vi "set print interval.vi"(4 "error in (no error)":errorcluster, 5 "auto/manual":bool, 6 "seconds/data point":u16=1 min=1 max=9999 step=1) -> (0 "error out":errorcluster, 2 "seconds/data point":u16=1 min=1 max=9999 step=1)   [LabVIEW 2010]
uses:
  serial commands.ctl
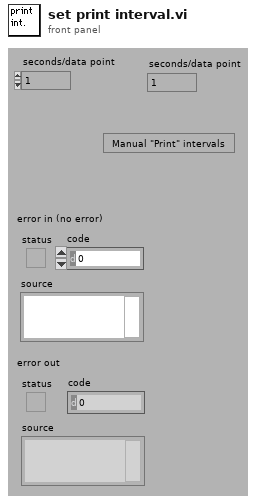
[diagram p1: front panel]
types:
  T1 = typedef "serial commands.ctl" = enum16{"configure", "VISA resource", "write line", "read line", "Clear buffer", "close"}
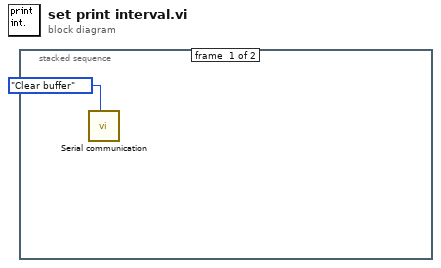
[diagram p0: block diagram]
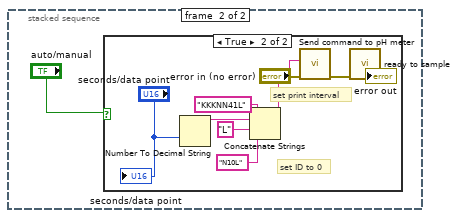
[diagram p2: hidden frame]
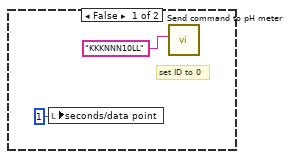
[diagram p3: hidden frame]
diagram:
  n1 = stacked-sequence {
    frame #0 {
      n2 = call <userlib>:"Serial communication.vi"("serial commands"=serial_commands."Clear buffer") -> ()  [unwired: 4 in, 4 out]
    }
    frame #1 {
      n3 = case shown="True" "auto/manual" {
        frame False {
          # "set ID to 0"
          n4 = local write "seconds/data point"(1) -> ()
          n5 = call "Send command to pH meter"("string to write"="KKKNNN10LL") -> ()  [unwired: 9 in, 2 out]
        }
        frame True {
          # "set print interval"
          # "set ID to 0"
          n6 = Number To Decimal String(number="seconds/data point") -> (decimal integer string=w11:string)  [unwired: 1 in]
          n7 = Concatenate Strings("KKKNN41L", w11, "L", "N10L") -> (w8:string)
          n8 = call "Send command to pH meter"("error in (no error)"="error in (no error)", "string to write"=w8) -> ("error out"=w7:errorcluster)  [unwired: 8 in, 1 out]
          n9 = call "ready to sample.vi"("error in (no error)"=w7) -> ("error out"=→"error out":errorcluster)  [unwired: 6 in]
          "seconds/data point" <- "seconds/data point"
        }
      }
    }
  }
